vi "Image File Dialog (Optional).vi"(6 "Dialog?":bool, 8 "Error In":errorcluster, 10 "Image File Format in":T1, 11 "Default file path in":path) -> (0 "Error Out":errorcluster, 2 "Image File Format out":T1, 3 "file path out":path)   [LabVIEW 2021, in "Image.lvlib"]
uses:
  Image Save File Format.ctl
  <vilib>/Utility/error.llb/Error Cluster From Error Code.vi
  <vilib>/ErrorRing/Error Ring.xnode
  Image.lvlib
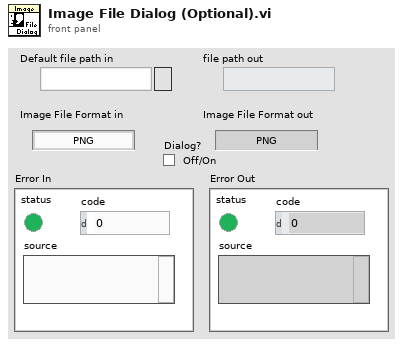
[diagram p1: front panel]
types:
  T1 = typedef "Image.lvlib/Image Save File Format.ctl" = enum16{"PNG", "JPEG", "BMP"}
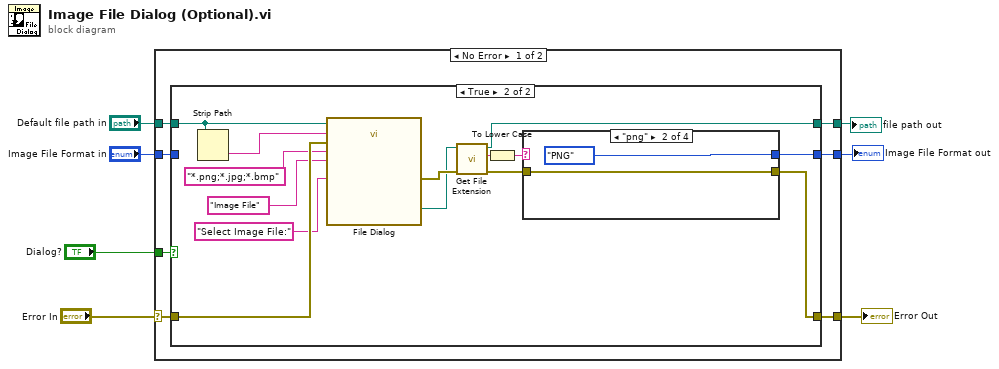
[diagram p0: block diagram]
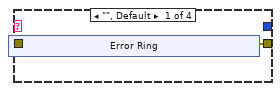
[diagram p3: hidden frame]
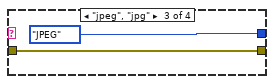
[diagram p4: hidden frame]
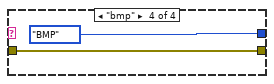
[diagram p5: hidden frame]
diagram:
  n1 = case shown="No Error" "Error In" {
    selector: "Error In" -> [w9 w43]
    tunnel: "Dialog?" -> [w14 _]
    tunnel: "Default file path in" -> [w13 w45]
    tunnel: [w12 w45] -> w5
    tunnel: "Image File Format in" -> [w11 w44]
    tunnel: [w10 w44] -> w3
    tunnel: [w8 w43] -> w1
    frame No Error {
      n2 = case shown="True" w14 {
        tunnel: w13 -> [w17 w30]
        tunnel: [w17 w23] -> w12
        tunnel: w11 -> [w16 _]
        tunnel: [w16 w19] -> w10
        tunnel: w9 -> [w15 w31]
        tunnel: [w15 w18] -> w8
        frame False {
        }
        frame True {
          n3 = Strip Path(path=w30) -> (name=w29:string)  [unwired: 1 out]
          n4 = call "File Dialog"("start path"=w30, "prompt"="Select Image File:", "default name"=w29, "error in"=w31, "pattern (all files)"="*.png;*.jpg;*.bmp", "pattern label"="Image File") -> ("selected path"=w24:path, "error out"=w25:errorcluster)  [unwired: 6 in, 2 out]
          n5 = call <vilib>:"Get File Extension.vi"("error in (no error)"=w25, "file"=w24) -> ("error out"=w21:errorcluster, "lowercase file extension"=w22:string, "dup file"=w23:path)  [unwired: 5 in, 2 out]
          n6 = To Lower Case(string=w22) -> (all lower case string=w20:string)
          n7 = case shown="\"png\"" w20 {
            tunnel: w21 -> [_ w37 w39 w41]
            tunnel: [_ Image_Save_File_Format."PNG" ("Image File Format in") Image_Save_File_Format."JPEG" ("Image File Format in") Image_Save_File_Format."BMP" ("Image File Format in")] -> w19
            tunnel: [w32 w37 w39 w41] -> w18
            frame "", Default {
              n8 = xnode "Error Ring"() -> ("error out"=w32:errorcluster)
            }
            frame "png" {
            }
            frame "jpeg", "jpg" {
            }
            frame "bmp" {
            }
          }
        }
      }
    }
    frame Error {
    }
  }
  "Image File Format out" <- w3
  "file path out" <- w5
  "Error Out" <- w1
